vi "HardwareLoop.vi"(8 "Error In":errorcluster, 10 "Data Structures":T1, 11 "Action Queues":T2) -> (0 "Error Out":errorcluster)   [LabVIEW 2012]
uses:
  ActionQueues.ctl
  UIActionQueueElement.ctl
  UIAction.ctl
  HardwareActionQueueElement.ctl
  HardwareAction.ctl
  HeaterActionQueueElement.ctl
  HeaterAction.ctl
  MFCActionQueueElement.ctl
  MFCAction.ctl
  LogActionQueueElement.ctl
  LogAction.ctl
  DataStructures.ctl
  HardwareDisplayData.ctl
  HardwareLogData.ctl
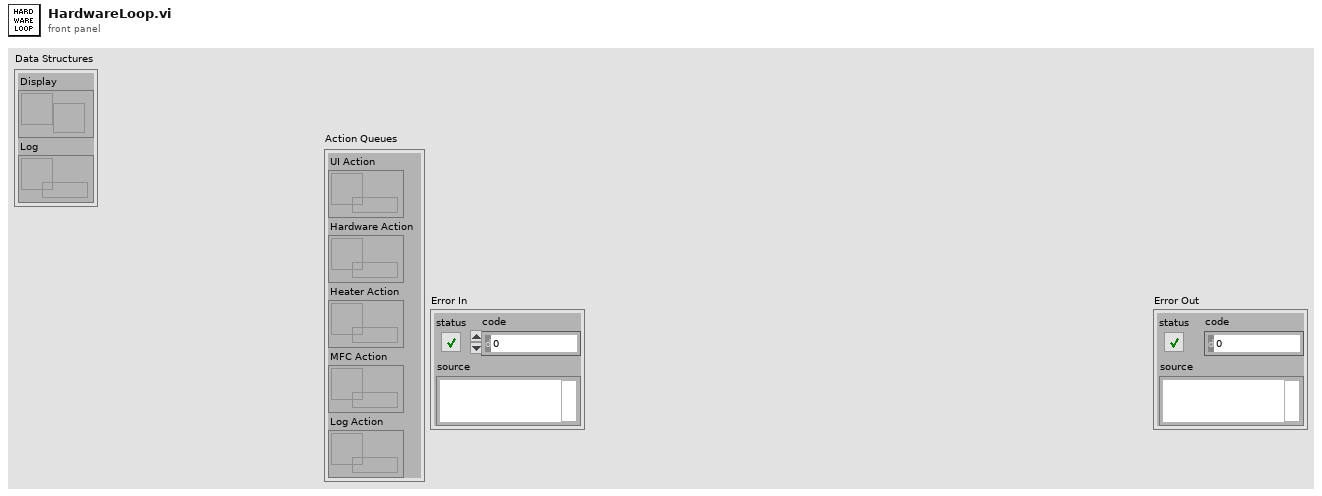
[diagram p1: front panel]
types:
  T1 = typedef "DataStructures.ctl" = cluster{"Display":refnum<notifier>, "Log":refnum<queue>}
  T2 = typedef "ActionQueues.ctl" = cluster{"UI Action":refnum<queue>, "Hardware Action":refnum<queue>, "Heater Action":refnum<queue>, "MFC Action":refnum<queue>, "Log Action":refnum<queue>}
  T3 = typedef "HardwareDataStructures.ctl" = cluster{"Heater":refnum<notifier>, "MFC":refnum<notifier>}
  T4 = typedef "HardwareDisplayData.ctl" = cluster{"Heater":dbl, "MFC":dbl}
  T5 = typedef "HardwareLogData.ctl" = cluster{"Timestamp":timestamp, "Data":T4}
  T6 = typedef "HardwareActionQueueElement.ctl" = cluster{"Action":T7, "Data":variant}
  T7 = typedef "HardwareAction.ctl" = enum16{"Initialize", "Collect", "Shutdown"}
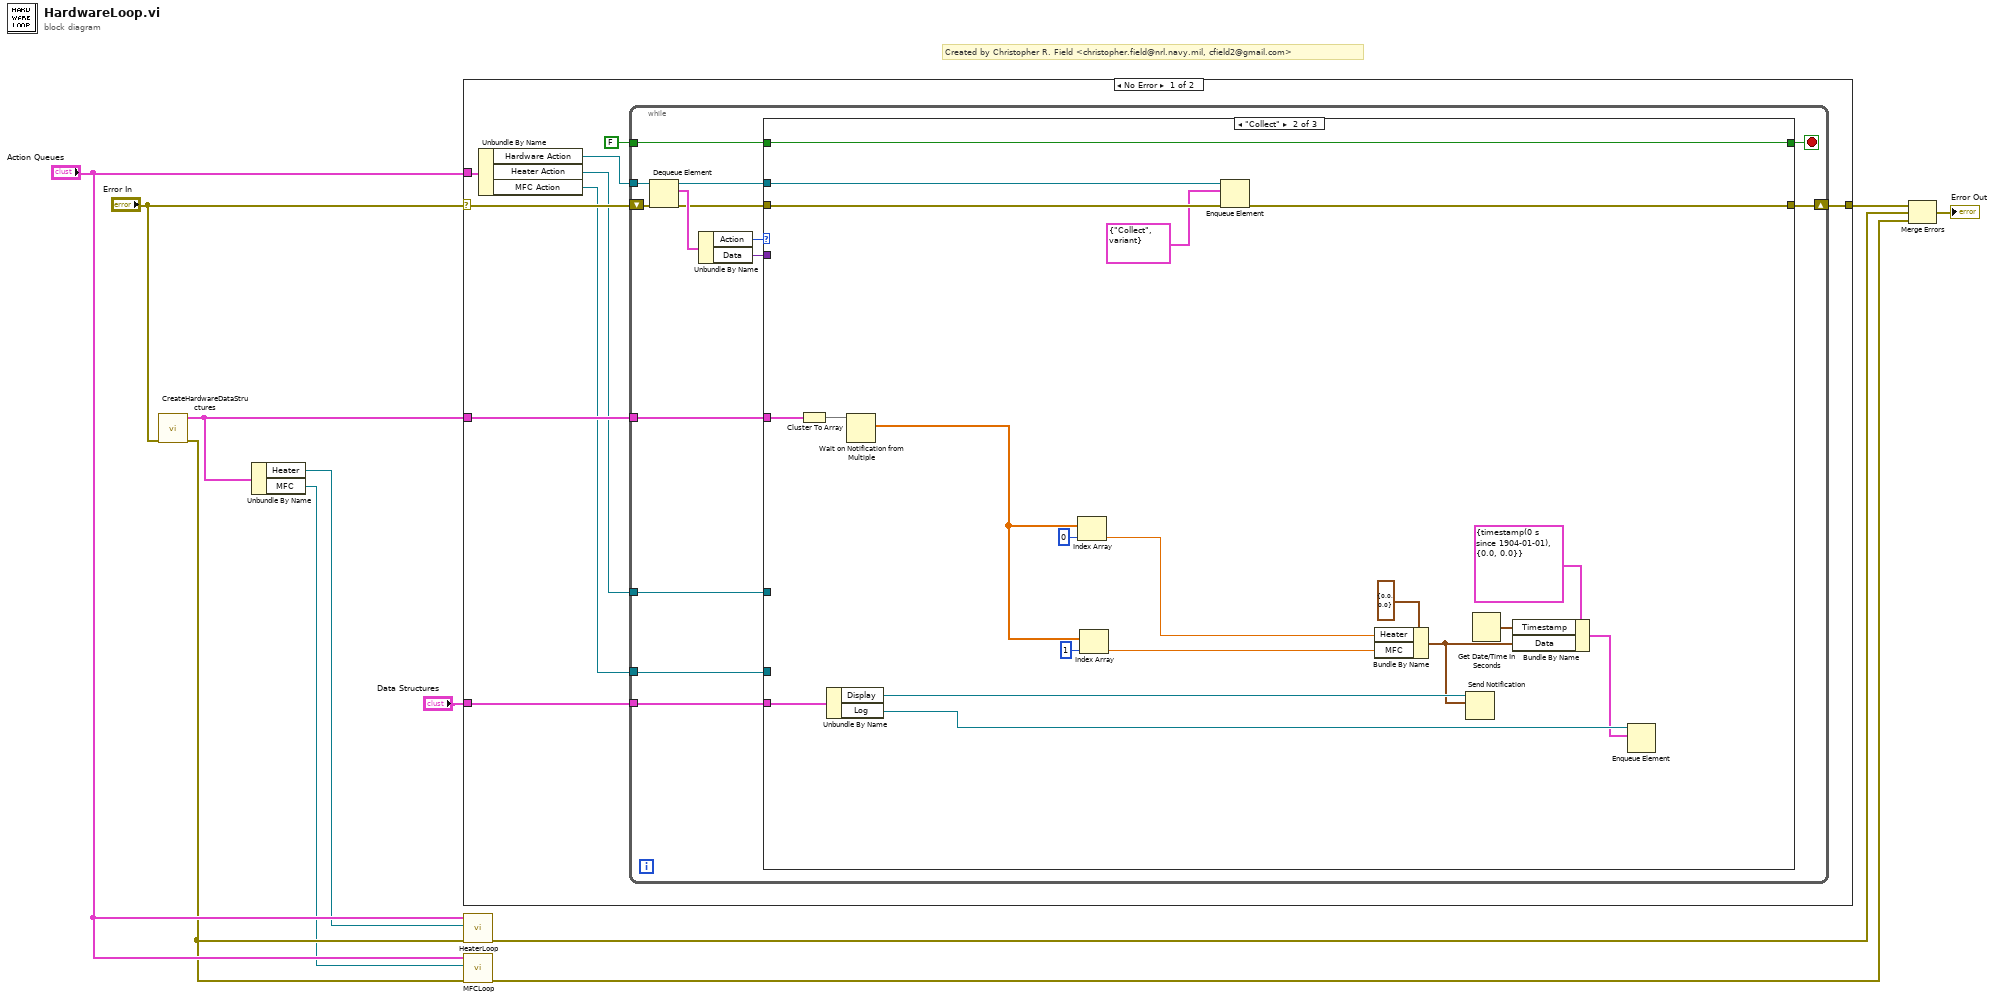
[diagram p0: block diagram]
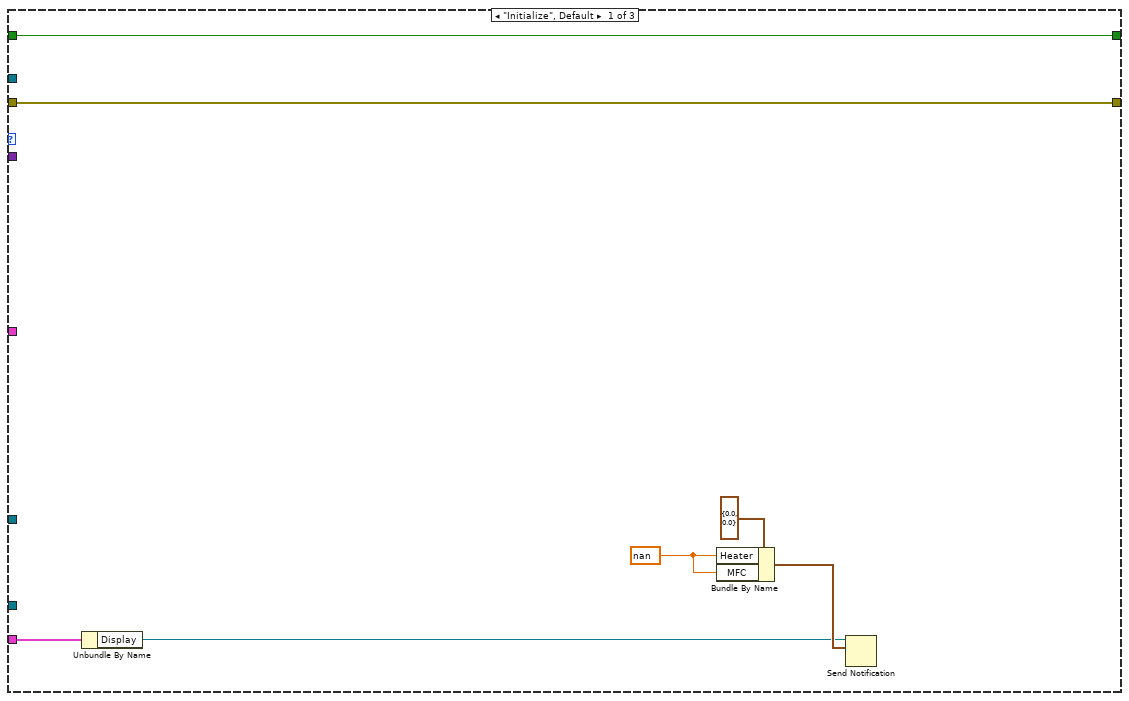
[diagram p2: hidden frame]
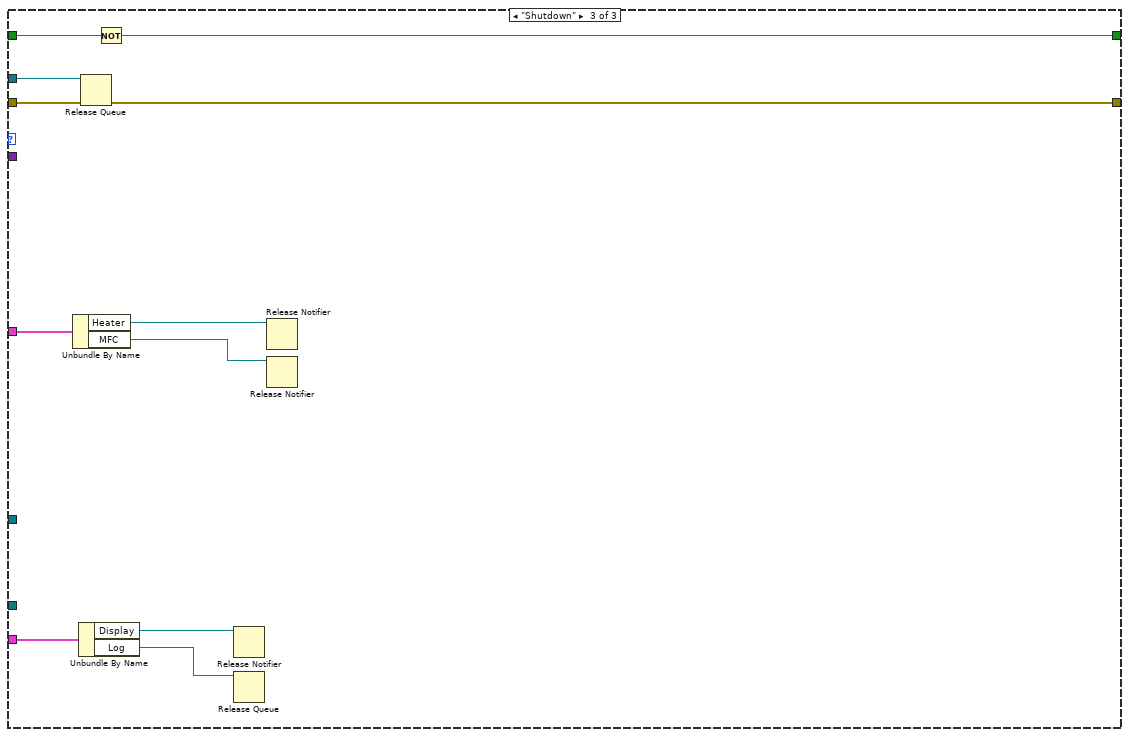
[diagram p3: hidden frame]
diagram:
  # "Created by Christopher R. Field <christopher.field@nrl.navy.mil, cfield2@gmail.com>"
  n1 = call "CreateHardwareDataStructures.vi"("Error In"="Error In") -> ("Error Out"=w3:errorcluster, "Hardware Data Structures"=w6:T3)  [unwired: 9 in]
  n2 = Unbundle By Name(w6) -> ("Heater"=w1:refnum<notifier>, "MFC"=w2:refnum<notifier>)
  n3 = case shown="No Error" "Error In" {
    selector: "Error In" -> [w16 w73]
    tunnel: [w19 w73] -> w11
    tunnel: "Action Queues" -> [w18 _]
    tunnel: "Data Structures" -> [w15 _]
    tunnel: w6 -> [w14 _]
    frame No Error {
      n4 = Unbundle By Name(w18) -> ("Hardware Action"=w17:refnum<queue>, "Heater Action"=w13:refnum<queue>, "MFC Action"=w12:refnum<queue>)
      n5 = while {
        tunnel: FALSE -> [w34]
        shift-right: [w27] -> w19
        shift-left: w16 -> [w33]
        tunnel: w17 -> [w25]
        tunnel: w14 -> [w24]
        tunnel: w15 -> [w23]
        tunnel: w13 -> [w22]
        tunnel: w12 -> [w21]
        stop <- w26 stop-if-true
        n6 = Dequeue Element(queue=w25, error in (no error)=w33) -> (queue out=w32:refnum<queue>, element=w31:T6, error out=w28:errorcluster)  [unwired: 1 in, 1 out]
        n7 = Unbundle By Name(w31) -> ("Action"=w30:T7, "Data"=w29:variant)
        n8 = case shown="\"Collect\"" w30 {
          tunnel: w34 -> [w41 w61 w72]
          tunnel: w32 -> [_ w60 w70]
          tunnel: w29 -> [_ _ _]
          tunnel: w28 -> [w40 w59 w69]
          tunnel: [w40 w58 w68] -> w27
          tunnel: [w41 w61 w71] -> w26
          tunnel: w24 -> [_ w48 w65]
          tunnel: w23 -> [w39 w55 w67]
          tunnel: w22 -> [_ _ _]
          tunnel: w21 -> [_ _ _]
          frame "Initialize", Default {
            w35 = nan ("Heater")
            n9 = Unbundle By Name(w39) -> ("Display"=w36:refnum<notifier>)
            n10 = Bundle By Name(cluster=T4 {"Heater"=0.0, "MFC"=0.0} ("Hardware Display Data"), "Heater"=w35, "MFC"=w35) -> (w37:T4)
            n11 = Send Notification(notification=w37, notifier=w36) -> ()  [unwired: 1 in, 2 out]
          }
          frame "Collect" {
            n12 = Cluster To Array(cluster=w48) -> (array=w47:refnum<notifier>[])
            n13 = Unbundle By Name(w55) -> ("Display"=w54:refnum<notifier>, "Log"=w53:refnum<queue>)
            n14 = Wait on Notification from Multiple(0:w47) -> (9:w44:dbl[])  [unwired: 3 in, 3 out]
            n15 = Index Array(array=w44, index=0) -> (element=w45:dbl)
            n16 = Index Array(array=w44, index=1) -> (element=w42:dbl)
            n17 = Enqueue Element(queue=w60, element=T6 {"Action"=enum."Collect", "Data"=variant}, error in (no error)=w59) -> (error out=w58:errorcluster)  [unwired: 1 in, 2 out]
            n18 = Bundle By Name(cluster=T4 {"Heater"=0.0, "MFC"=0.0} ("Hardware Display Data"), "Heater"=w45, "MFC"=w42) -> (w50:T4)
            n19 = Send Notification(notification=w50, notifier=w54) -> ()  [unwired: 1 in, 2 out]
            n20 = Get Date/Time In Seconds() -> (seconds since 1Jan1904=w51:timestamp)
            n21 = Bundle By Name(cluster=T5 {"Timestamp"=timestamp(0 s since 1904-01-01), "Data"={"Heater"=0.0, "MFC"=0.0}} ("Hardware Log Data"), "Timestamp"=w51, "Data"=w50) -> (w49:T5)
            n22 = Enqueue Element(queue=w53, element=w49) -> ()  [unwired: 2 in, 3 out]
          }
          frame "Shutdown" {
            n23 = Unbundle By Name(w65) -> ("Heater"=w64:refnum<notifier>, "MFC"=w63:refnum<notifier>)
            n24 = Unbundle By Name(w67) -> ("Display"=w66:refnum<notifier>, "Log"=w62:refnum<queue>)
            n25 = Release Queue(queue=w70, error in (no error)=w69) -> (error out=w68:errorcluster)  [unwired: 1 in, 2 out]
            n26 = Not(x=w72) -> (.not. x?=w71:bool)
            n27 = Release Notifier(notifier=w66) -> ()  [unwired: 2 in, 3 out]
            n28 = Release Queue(queue=w62) -> ()  [unwired: 2 in, 3 out]
            n29 = Release Notifier(notifier=w64) -> ()  [unwired: 2 in, 3 out]
            n30 = Release Notifier(notifier=w63) -> ()  [unwired: 2 in, 3 out]
          }
        }
      }
    }
    frame Error {
    }
  }
  n31 = call "HeaterLoop.vi"("Error In"=w3, "Heater Data"=w1, "Action Queues"="Action Queues") -> ("Error Out"=w8:errorcluster)  [unwired: 8 in]
  n32 = call "MFCLoop.vi"("Error In"=w3, "MFC Data"=w2, "Action Queues"="Action Queues") -> ("Error Out"=w7:errorcluster)  [unwired: 8 in]
  n33 = Merge Errors(w11, w8, w7) -> (→"Error Out":errorcluster)
